vi "ZLIB Open Unzip Archive__ogtk.vi"(4 "error in (no error)":errorcluster, 7 "archive name":path) -> (0 "error out":errorcluster, 3 "unzip Refnum":T1)   [LabVIEW 2014]
doc: "Opens an unzip session."
uses:
  ZLIB Unzip Handle__ogtk.ctl
  <userlib>/_OpenG.lib/lvzip/lvzlib.dll
panel:
  # "Please visit http://www.OpenG.org to learn about the\nOpen Source LabVIEW software movement.\n\nNOTICE -- YOU MUST LEAVE THIS NOTICE IN PLACE.  PER THE TERMS OF THE LICENSE BELOW, YOU MAY SUBLICENSE THIS SOFTWARE \nIN ANY WAY THAT DOES NOT CONFLICT WITH THIS LICENSE.\n\n### BSD License (http://www.opensource.org/licenses/bsd-license.php) Begin ###\n \nCopyright (C) 2002-2004 Rolf Kalbermatter rolf.kalbermatter@citeng.com\nCopyright (C) 2002 Jim Kring jim@jimkring.com\n\nAll rights reserved.\n\nRedistribution and use in source and binary forms, with or without modification, are permitted provided that the following conditions are met:\n\n    * Redistributions of source code must retain the above copyright notice, this list of conditions and the following disclaimer.\n    * Redistributions in binary form must reproduce the above copyright notice, this list of conditions and the following disclaimer in the \n       documentation and/or other materials provided with the distribution.\n    * Neither the name of SciWare, James Kring, Inc., nor the names of its contributors may be used to endorse or promote products derived \n       from this software without specific prior written permission.\n\nTHIS SOFTWARE IS PROVIDED BY THE COPYRIGHT HOLDERS AND CONTRIBUTORS \"AS IS\" AND ANY EXPRESS OR IMPLIED WARRANTIES, \nINCLUDING, BUT NOT LIMITED TO, THE IMPLIED WARRANTIES OF MERCHANTABILITY AND FITNESS FOR A PARTICULAR PURPOSE ARE \nDISCLAIMED. IN NO EVENT SHALL THE COPYRIGHT OWNER OR CONTRIBUTORS BE LIABLE FOR ANY DIRECT, INDIRECT, INCIDENTAL,\n SPECIAL, EXEMPLARY, OR CONSEQUENTIAL DAMAGES (INCLUDING, BUT NOT LIMITED TO, PROCUREMENT OF SUBSTITUTE GOODS OR \nSERVICES; LOSS OF USE, DATA, OR PROFITS; OR BUSINESS INTERRUPTION) HOWEVER CAUSED AND ON ANY THEORY OF LIABILITY, \nWHETHER IN CONTRACT, STRICT LIABILITY, OR TORT (INCLUDING NEGLIGENCE OR OTHERWISE) ARISING IN ANY WAY OUT OF THE USE \nOF THIS SOFTWARE, EVEN IF ADVISED OF THE POSSIBILITY OF SUCH DAMAGE.\n\n### BSD License End ###"
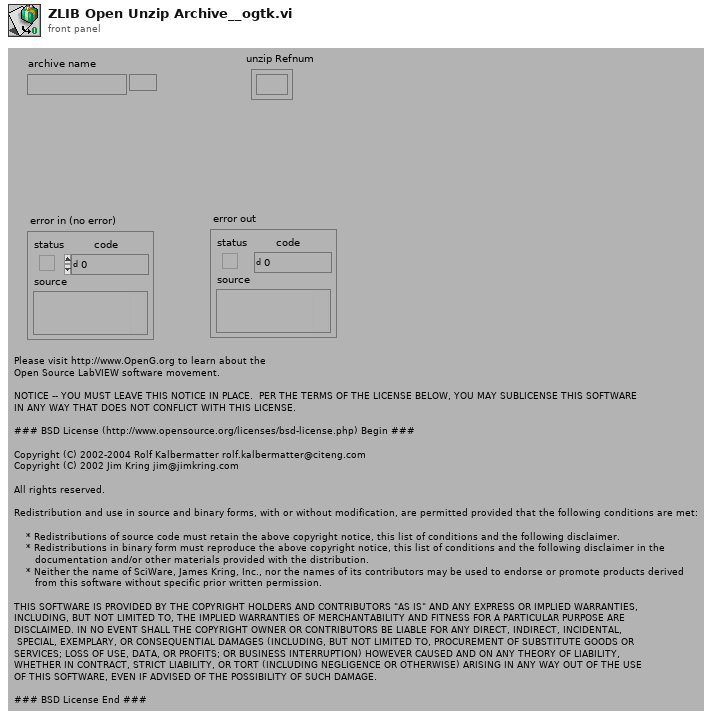
[diagram p1: front panel]
types:
  T1 = typedef "ZLIB Unzip Handle__ogtk.ctl" = refnum<k1>
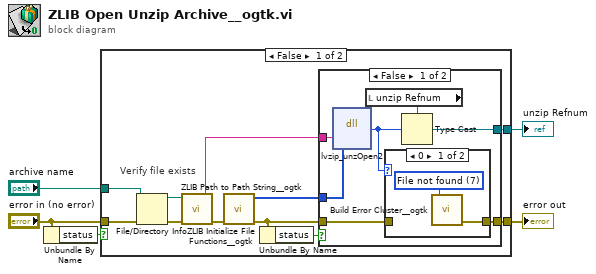
[diagram p0: block diagram]
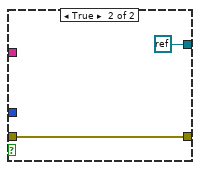
[diagram p3: hidden frame]
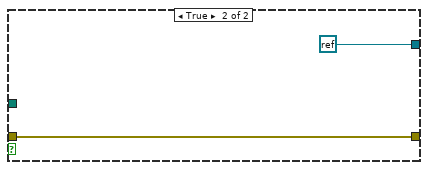
[diagram p4: hidden frame]
diagram:
  n1 = Unbundle By Name("error in (no error)") -> ("status"=w2:bool)
  n2 = case shown="False" w2 {
    tunnel: "archive name" -> [w8 _]
    tunnel: [w16 refnum<k0> refnum] -> w4
    tunnel: "error in (no error)" -> [w7 w29]
    tunnel: [w15 w29] -> w1
    frame False {
      # "Verify file exists"
      n3 = File/Directory Info(path=w8, error in=w7) -> (path out=w14:path, error out=w6:errorcluster)  [unwired: 5 out]
      n4 = call "ZLIB Path to Path String__ogtk.vi"("error in (no error)"=w6, "LV file path"=w14) -> ("error in (no error)"=w12:errorcluster, "path string"=w13:string)  [unwired: 4 in]
      n5 = call "ZLIB Initialize File Functions__ogtk.vi"("error in (no error)"=w12) -> ("error out"=w10:errorcluster, "fileFuncs"=w11:u8[])  [unwired: 5 in]
      n6 = Unbundle By Name(w10) -> ("status"=w9:bool)
      n7 = case shown="False" w9 {
        tunnel: [w22 refnum<k0> refnum] -> w16
        tunnel: [w20 w27] -> w15
        tunnel: w13 -> [w19 _]
        tunnel: w10 -> [w18 w27]
        tunnel: w11 -> [w17 _]
        frame False {
          n8 = dll-call lib="C:/Program Files/National Instruments/LabVIEW 2014/user.lib/_OpenG.lib/lvzip/lvzlib.*" fn="lvzip_unzOpen2"("path"=w19, "fileFuncs"=w17) -> (w23:u32)  [unwired: 5 in, 2 out]
          n9 = local read "unzip Refnum"() -> (w21:T1)
          n10 = case shown="0" w23 {
            tunnel: w18 -> [_ w26]
            tunnel: [w25 w26] -> w20
            frame 0 {
              w24 = 7 items=["No error", "Argument error", "Memory is full", "Out of zone", "End of file", "File already open", "Generic file I/O error", "File not found", "File permission error", "Disk is full", "Duplicate path", "Too many files open", "System feature not enabled", "Resource file not found", "Cannot add resource", "Resource not found", "Image not found", "Image memory error", "Pen does not exist", "Config type invalid", "Config token not found", "Config parse error", "Config memory error", "Bad external code format", "Bad external code offset", "External code not present", "Null window", "Destroy window error", "Null menu", "Print aborted", "Bad print record", "Print driver error", "Windows error during printing", "Memory error during printing", "Print dialog error", "Generic print error", "Invalid device refnum", "Device not found", "Device parameter error", "Device unit error", "Cannot open device", "Device call aborted", "Generic error", "Cancelled by user", "Object ID too low", "Object ID too high", "Object not in heap", "Unknown heap", "Unknown object (invalid DefProc)", "Unknown object (DefProc not in table)", "Message out of range", "Invalid (null) method", "Unknown message", "Manager call not supported", "Bad address", "Network operation in progress", "Network operation timed out", "Connection is busy", "Network attribute not supported", "Network error", "Address in use", "System out of memory", "Connection aborted", "Connection refused", "Not connected", "Already connected", "Connection closed", "Initialization error (interapplication manager)", "Bad occurrence", "Wait on unbound occurrence handler", "Occurrence queue overflow", "Datalog type conflict", "Unused", "Unrecognized type (interapplication manager)", "Memory corrupt", "Failed to make temporary DLL", "Old CIN version", "Drag socket not found", "Failed to load drop-object", "Failed to register OLE object", "Failed to release OLE object", "Format specifier type mismatch", "Unknown format specifier", "Too few format specifiers", "Too many format specifiers", "Scan failed", "Newer CIN version", "Error converting to variant", "Runtime menu error", "Password tampered", "Variant attribute not found", "Incompatible variant data type", "Event data is not available", "Event Store is not present", "Occurrence is not found", "Event Queue is not created", "Event info is not available", "Refnum passed is NULL", "Error retrieving Class GUID", "Error retrieving CoClass GUID", "Error retrieving TypeLib GUID.", "Bad built application magic bytes.", "Specific driver is different from the specific driver associated with the Logical Name.", "There is no session opened to the class driver.", "Max Error", "MAX - Error with config objects", "MAX - Error loading configuration", "MAX - Group not supported"]
              n11 = call "Build Error Cluster__ogtk.vi"("code"=w24) -> ("error out"=w25:errorcluster)  [unwired: 1 in]
            }
            frame Default {
            }
          }
          n12 = Type Cast(type=w21, x=w23) -> (*(type *) &x=w22:T1)
        }
        frame True {
        }
      }
    }
    frame True {
    }
  }
  "error out" <- w1
  "unzip Refnum" <- w4
